vi "Add Device.vi"(8 "error in (no error)":errorcluster, 11 "Node Ptr":u64 format="%.0x") -> (0 "error out":errorcluster)   [LabVIEW 2010, in "PXIe-433x Custom Device.lvlib"]
uses:
  PXIe-433x Custom Device.lvlib
  Global.vi
  <vilib>/NI Veristand/Custom Device API/Custom Device API.lvlib
panel:
  in  "Tag":string
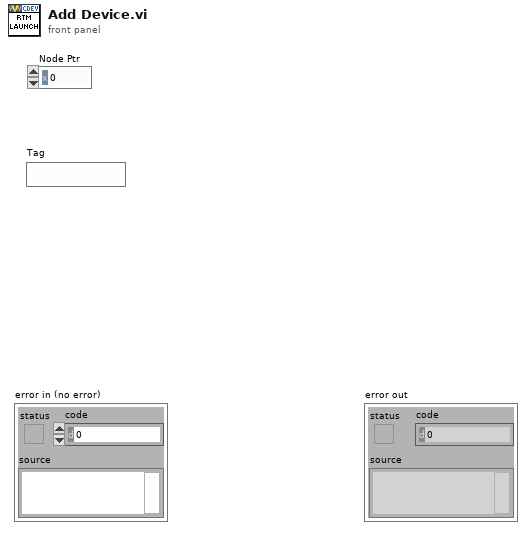
[diagram p1: front panel]
types:
  T1 = typedef "Custom Device API.lvlib/Custom Device Item Ref.ctl" = u64
  T2 = typedef "PXIe-433x Custom Device.lvlib/Max Value.ctl" = dbl
  T3 = typedef "PXIe-433x Custom Device.lvlib/Sensor Type.ctl" = enum16{"Strain", "Force", "Pressure", "Torque"}
  T4 = typedef "PXIe-433x Custom Device.lvlib/Min Value.ctl" = dbl
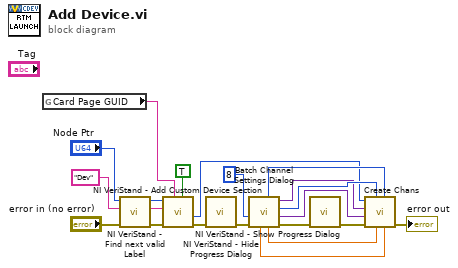
[diagram p0: block diagram]
diagram:
  n1 = global read "Global.vi" "Card Page GUID"() -> (w16:string)
  n2 = call <vilib>:"NI VeriStand - Find next valid Label.vi"("error in (no error)"="error in (no error)", "Label"="Dev", "Item Ref in"="Node Ptr") -> ("error out"=w12:errorcluster, "Label out"=w13:string, "Item Ref out"=w14:T1)  [unwired: 4 in, 2 out]
  n3 = call <vilib>:"NI VeriStand - Add Custom Device Section.vi"("Highlight? (F)"=TRUE, "GUID (Default Section)"=w16, "error in (no error)"=w12, "Section Name"=w13, "Parent Ref in"=w14) -> ("error out"=w2:errorcluster, "Section Ptr"=w3:T1)  [unwired: 3 in, 2 out]
  n4 = call <vilib>:"NI VeriStand - Hide Progress Dialog.vi"("error in (no error)"=w2) -> ("error out"=w6:errorcluster)  [unwired: 10 in]
  n5 = call "Batch Channel Settings Dialog.vi"("error in (no error)"=w6, "Data Entry Limits:Maximum"=8) -> ("error out"=w5:errorcluster, "scaling information"=w18:variant, "# of Chans"=w20:u8, "bridge information"=w19:variant, "Maximum Value"=w21:T2, "Sensor Type"=w17:T3, "Minimum Value"=w9:T4)  [unwired: 3 in]
  n6 = call <vilib>:"NI VeriStand - Show Progress Dialog.vi"("error in (no error)"=w5) -> ("error out"=w4:errorcluster)  [unwired: 10 in]
  n7 = call "Create Chans.vi"("Minimum Value"=w9, "Sensor Type"=w17, "Maximum Value"=w21, "# of Chans"=w20, "error in"=w4, "scaling information"=w18, "bridge information"=w19, "Item Ref in"=w3) -> ("error out"=→"error out":errorcluster)  [unwired: 2 in, 1 out]
